vi "Legacy-monitor.vi"() -> ()   [LabVIEW 2016]
uses:
  controls/SCA states.ctl
panel:
  out "Start Sample Change":bool
  out "Rotate Wheel":bool
  out "Venting Source":bool
  out "Pumping out Source":bool
  out "insert Retract Rod":bool
  out "retract Retract Rod":bool
  out "Open Wheel GV":bool
  out "Close Wheel GV":bool
  out "insert Insert Rod":bool
  out "retract Insert Rod":bool
  out "insert Sample Rod":bool
  out "retract Sample Rod":bool
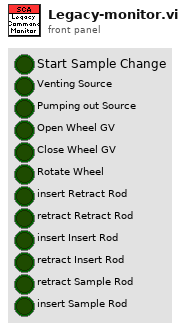
[diagram p1: front panel]
types:
  T1 = typedef "SCA states.ctl" = enum16{"initialize", "wait", "change sample start", "change sample", "check position", "rotate wheel", "sample change complete", "sample rod up", "sample rod down", "retract rod in", "retract rod out", "insert rod in", "insert rod out", "wheel GV open", "wheel GV close", "vent source", "pump source", "shutdown"}
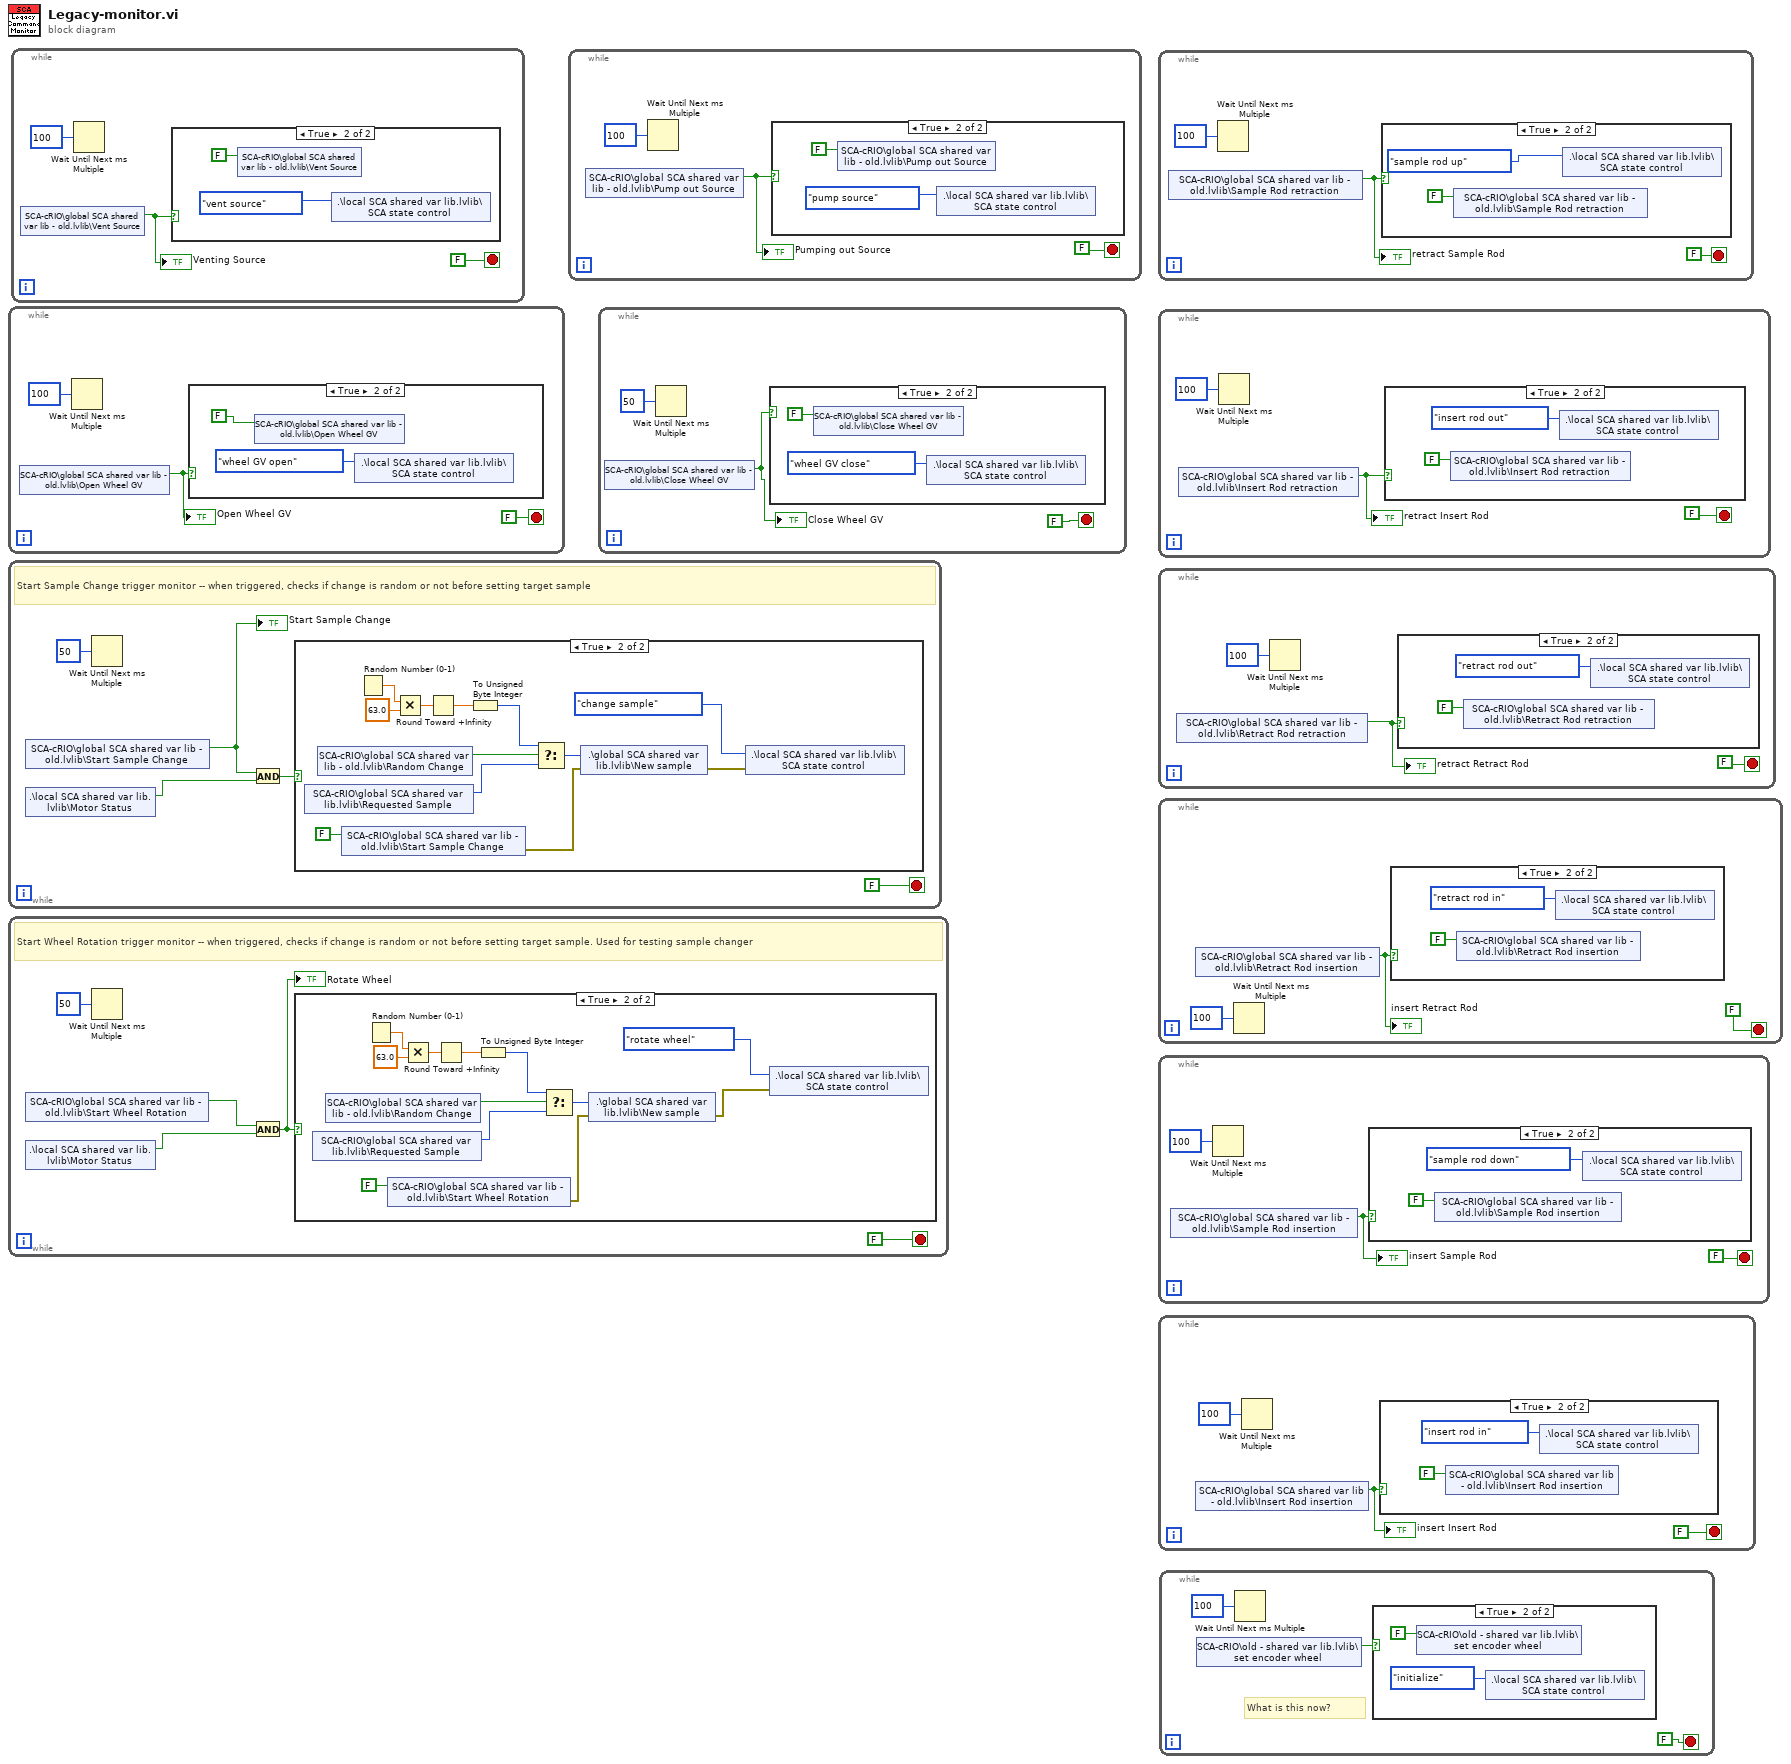
[diagram p0: block diagram]
diagram:
  n1 = while {
    stop <- FALSE stop-if-true
    n2 = shared-variable "SCA-cRIO\\global SCA shared var lib - old.lvlib\\Open Wheel GV"() -> (w2:bool)  [unwired: 1 in, 1 out]
    "Open Wheel GV" <- w2
    n3 = Wait Until Next ms Multiple(millisecond multiple=u32 100) -> ()  [unwired: 1 out]
    n4 = case shown="True" w2 {
      frame False {
      }
      frame True {
        n5 = shared-variable "SCA-cRIO\\global SCA shared var lib - old.lvlib\\Open Wheel GV"(FALSE ("rod up shared")) -> ()  [unwired: 1 in, 1 out]
        n6 = shared-variable ".\\local SCA shared var lib.lvlib\\SCA state control"(SCA_states."wheel GV open" ("SC2 state")) -> ()  [unwired: 1 in, 1 out]
      }
    }
  }
  n7 = while {
    stop <- FALSE stop-if-true
    # "Start Sample Change trigger monitor -- when triggered, checks if change is random or not before setting target sample"
    n8 = shared-variable "SCA-cRIO\\global SCA shared var lib - old.lvlib\\Start Sample Change"() -> (w8:bool)  [unwired: 1 in, 1 out]
    "Start Sample Change" <- w8
    n9 = shared-variable ".\\local SCA shared var lib.lvlib\\Motor Status"() -> (w6:bool)  [unwired: 1 in, 1 out]
    n10 = Wait Until Next ms Multiple(millisecond multiple=u32 50) -> ()  [unwired: 1 out]
    n11 = And(x=w8, y=w6) -> (x .and. y?=w7:bool)
    n12 = case shown="True" w7 {
      frame False {
      }
      frame True {
        n13 = shared-variable "SCA-cRIO\\global SCA shared var lib.lvlib\\Requested Sample"() -> (w14:u8)  [unwired: 1 in, 1 out]
        n14 = shared-variable "SCA-cRIO\\global SCA shared var lib - old.lvlib\\Random Change"() -> (w13:bool)  [unwired: 1 in, 1 out]
        n15 = shared-variable "SCA-cRIO\\global SCA shared var lib - old.lvlib\\Start Sample Change"(FALSE ("rod up shared")) -> (error out=w11:errorcluster)  [unwired: 1 in]
        n16 = Random Number (0-1)() -> (number: 0 to 1=w18:dbl)
        n17 = Multiply(x=w18, y=63.0) -> (x*y=w16:dbl)
        n18 = Round Toward +Infinity(x=w16) -> (ceil(x): smallest int >= x=w19:dbl)
        n19 = To Unsigned Byte Integer(number=w19) -> (unsigned 8bit integer=w20:u8)
        n20 = Select(t=w20, s=w13, f=w14) -> (s? t:f=w15:u8)
        n21 = shared-variable ".\\global SCA shared var lib.lvlib\\New sample"(w15, error in=w11) -> (error out=w12:errorcluster)
        n22 = shared-variable ".\\local SCA shared var lib.lvlib\\SCA state control"(SCA_states."change sample" ("SC2 state"), error in=w12) -> ()  [unwired: 1 out]
      }
    }
  }
  n23 = while {
    stop <- FALSE stop-if-true
    # "Start Wheel Rotation trigger monitor -- when triggered, checks if change is random or not before setting target sample. Used for testing sample changer"
    n24 = shared-variable "SCA-cRIO\\global SCA shared var lib - old.lvlib\\Start Wheel Rotation"() -> (w25:bool)  [unwired: 1 in, 1 out]
    n25 = shared-variable ".\\local SCA shared var lib.lvlib\\Motor Status"() -> (w24:bool)  [unwired: 1 in, 1 out]
    n26 = Wait Until Next ms Multiple(millisecond multiple=u32 50) -> ()  [unwired: 1 out]
    n27 = And(x=w25, y=w24) -> (x .and. y?=w23:bool)
    "Rotate Wheel" <- w23
    n28 = case shown="True" w23 {
      frame False {
      }
      frame True {
        n29 = shared-variable "SCA-cRIO\\global SCA shared var lib.lvlib\\Requested Sample"() -> (w31:u8)  [unwired: 1 in, 1 out]
        n30 = shared-variable "SCA-cRIO\\global SCA shared var lib - old.lvlib\\Random Change"() -> (w30:bool)  [unwired: 1 in, 1 out]
        n31 = Random Number (0-1)() -> (number: 0 to 1=w35:dbl)
        n32 = shared-variable "SCA-cRIO\\global SCA shared var lib - old.lvlib\\Start Wheel Rotation"(FALSE ("rod up shared")) -> (error out=w28:errorcluster)  [unwired: 1 in]
        n33 = Multiply(x=w35, y=63.0) -> (x*y=w33:dbl)
        n34 = Round Toward +Infinity(x=w33) -> (ceil(x): smallest int >= x=w36:dbl)
        n35 = To Unsigned Byte Integer(number=w36) -> (unsigned 8bit integer=w37:u8)
        n36 = Select(t=w37, s=w30, f=w31) -> (s? t:f=w32:u8)
        n37 = shared-variable ".\\global SCA shared var lib.lvlib\\New sample"(w32, error in=w28) -> (error out=w29:errorcluster)
        n38 = shared-variable ".\\local SCA shared var lib.lvlib\\SCA state control"(SCA_states."rotate wheel" ("SC2 state"), error in=w29) -> ()  [unwired: 1 out]
      }
    }
  }
  n39 = while {
    stop <- FALSE stop-if-true
    n40 = shared-variable "SCA-cRIO\\global SCA shared var lib - old.lvlib\\Vent Source"() -> (w41:bool)  [unwired: 1 in, 1 out]
    "Venting Source" <- w41
    n41 = Wait Until Next ms Multiple(millisecond multiple=u32 100) -> ()  [unwired: 1 out]
    n42 = case shown="True" w41 {
      frame False {
      }
      frame True {
        n43 = shared-variable "SCA-cRIO\\global SCA shared var lib - old.lvlib\\Vent Source"(FALSE ("rod up shared")) -> ()  [unwired: 1 in, 1 out]
        n44 = shared-variable ".\\local SCA shared var lib.lvlib\\SCA state control"(SCA_states."vent source" ("SCA state control")) -> ()  [unwired: 1 in, 1 out]
      }
    }
  }
  n45 = while {
    stop <- FALSE stop-if-true
    n46 = shared-variable "SCA-cRIO\\global SCA shared var lib - old.lvlib\\Pump out Source"() -> (w46:bool)  [unwired: 1 in, 1 out]
    "Pumping out Source" <- w46
    n47 = Wait Until Next ms Multiple(millisecond multiple=u32 100) -> ()  [unwired: 1 out]
    n48 = case shown="True" w46 {
      frame False {
      }
      frame True {
        n49 = shared-variable "SCA-cRIO\\global SCA shared var lib - old.lvlib\\Pump out Source"(FALSE ("rod up shared")) -> ()  [unwired: 1 in, 1 out]
        n50 = shared-variable ".\\local SCA shared var lib.lvlib\\SCA state control"(SCA_states."pump source" ("SCA state control")) -> ()  [unwired: 1 in, 1 out]
      }
    }
  }
  n51 = while {
    stop <- FALSE stop-if-true
    n52 = shared-variable "SCA-cRIO\\global SCA shared var lib - old.lvlib\\Close Wheel GV"() -> (w50:bool)  [unwired: 1 in, 1 out]
    "Close Wheel GV" <- w50
    n53 = Wait Until Next ms Multiple(millisecond multiple=u32 50) -> ()  [unwired: 1 out]
    n54 = case shown="True" w50 {
      frame False {
      }
      frame True {
        n55 = shared-variable "SCA-cRIO\\global SCA shared var lib - old.lvlib\\Close Wheel GV"(FALSE ("rod up shared")) -> ()  [unwired: 1 in, 1 out]
        n56 = shared-variable ".\\local SCA shared var lib.lvlib\\SCA state control"(SCA_states."wheel GV close" ("SC2 state")) -> ()  [unwired: 1 in, 1 out]
      }
    }
  }
  n57 = while {
    stop <- FALSE stop-if-true
    n58 = shared-variable "SCA-cRIO\\global SCA shared var lib - old.lvlib\\Sample Rod retraction"() -> (w56:bool)  [unwired: 1 in, 1 out]
    "retract Sample Rod" <- w56
    n59 = Wait Until Next ms Multiple(millisecond multiple=u32 100) -> ()  [unwired: 1 out]
    n60 = case shown="True" w56 {
      frame False {
      }
      frame True {
        n61 = shared-variable "SCA-cRIO\\global SCA shared var lib - old.lvlib\\Sample Rod retraction"(FALSE ("rod up shared")) -> ()  [unwired: 1 in, 1 out]
        n62 = shared-variable ".\\local SCA shared var lib.lvlib\\SCA state control"(SCA_states."sample rod up" ("SCA state control")) -> ()  [unwired: 1 in, 1 out]
      }
    }
  }
  n63 = while {
    stop <- FALSE stop-if-true
    n64 = shared-variable "SCA-cRIO\\global SCA shared var lib - old.lvlib\\Insert Rod retraction"() -> (w61:bool)  [unwired: 1 in, 1 out]
    "retract Insert Rod" <- w61
    n65 = Wait Until Next ms Multiple(millisecond multiple=u32 100) -> ()  [unwired: 1 out]
    n66 = case shown="True" w61 {
      frame False {
      }
      frame True {
        n67 = shared-variable "SCA-cRIO\\global SCA shared var lib - old.lvlib\\Insert Rod retraction"(FALSE ("rod up shared")) -> ()  [unwired: 1 in, 1 out]
        n68 = shared-variable ".\\local SCA shared var lib.lvlib\\SCA state control"(SCA_states."insert rod out" ("SC2 state")) -> ()  [unwired: 1 in, 1 out]
      }
    }
  }
  n69 = while {
    stop <- FALSE stop-if-true
    n70 = shared-variable "SCA-cRIO\\global SCA shared var lib - old.lvlib\\Retract Rod retraction"() -> (w66:bool)  [unwired: 1 in, 1 out]
    "retract Retract Rod" <- w66
    n71 = Wait Until Next ms Multiple(millisecond multiple=u32 100) -> ()  [unwired: 1 out]
    n72 = case shown="True" w66 {
      frame False {
      }
      frame True {
        n73 = shared-variable "SCA-cRIO\\global SCA shared var lib - old.lvlib\\Retract Rod retraction"(FALSE ("rod up shared")) -> ()  [unwired: 1 in, 1 out]
        n74 = shared-variable ".\\local SCA shared var lib.lvlib\\SCA state control"(SCA_states."retract rod out" ("SC2 state")) -> ()  [unwired: 1 in, 1 out]
      }
    }
  }
  n75 = while {
    stop <- FALSE stop-if-true
    n76 = shared-variable "SCA-cRIO\\global SCA shared var lib - old.lvlib\\Retract Rod insertion"() -> (w71:bool)  [unwired: 1 in, 1 out]
    "insert Retract Rod" <- w71
    n77 = Wait Until Next ms Multiple(millisecond multiple=u32 100) -> ()  [unwired: 1 out]
    n78 = case shown="True" w71 {
      frame False {
      }
      frame True {
        n79 = shared-variable "SCA-cRIO\\global SCA shared var lib - old.lvlib\\Retract Rod insertion"(FALSE ("rod up shared")) -> ()  [unwired: 1 in, 1 out]
        n80 = shared-variable ".\\local SCA shared var lib.lvlib\\SCA state control"(SCA_states."retract rod in" ("SC2 state")) -> ()  [unwired: 1 in, 1 out]
      }
    }
  }
  n81 = while {
    stop <- FALSE stop-if-true
    n82 = shared-variable "SCA-cRIO\\global SCA shared var lib - old.lvlib\\Sample Rod insertion"() -> (w76:bool)  [unwired: 1 in, 1 out]
    "insert Sample Rod" <- w76
    n83 = Wait Until Next ms Multiple(millisecond multiple=u32 100) -> ()  [unwired: 1 out]
    n84 = case shown="True" w76 {
      frame False {
      }
      frame True {
        n85 = shared-variable "SCA-cRIO\\global SCA shared var lib - old.lvlib\\Sample Rod insertion"(FALSE ("rod up shared")) -> ()  [unwired: 1 in, 1 out]
        n86 = shared-variable ".\\local SCA shared var lib.lvlib\\SCA state control"(SCA_states."sample rod down" ("SC2 state")) -> ()  [unwired: 1 in, 1 out]
      }
    }
  }
  n87 = while {
    stop <- FALSE stop-if-true
    n88 = shared-variable "SCA-cRIO\\global SCA shared var lib - old.lvlib\\Insert Rod insertion"() -> (w81:bool)  [unwired: 1 in, 1 out]
    "insert Insert Rod" <- w81
    n89 = Wait Until Next ms Multiple(millisecond multiple=u32 100) -> ()  [unwired: 1 out]
    n90 = case shown="True" w81 {
      frame False {
      }
      frame True {
        n91 = shared-variable "SCA-cRIO\\global SCA shared var lib - old.lvlib\\Insert Rod insertion"(FALSE ("rod up shared")) -> ()  [unwired: 1 in, 1 out]
        n92 = shared-variable ".\\local SCA shared var lib.lvlib\\SCA state control"(SCA_states."insert rod in" ("SC2 state")) -> ()  [unwired: 1 in, 1 out]
      }
    }
  }
  n93 = while {
    stop <- FALSE stop-if-true
    # "What is this now?"
    n94 = shared-variable "SCA-cRIO\\old - shared var lib.lvlib\\set encoder wheel"() -> (w85:bool)  [unwired: 1 in, 1 out]
    n95 = Wait Until Next ms Multiple(millisecond multiple=u32 100) -> ()  [unwired: 1 out]
    n96 = case shown="True" w85 {
      frame False {
      }
      frame True {
        n97 = shared-variable "SCA-cRIO\\old - shared var lib.lvlib\\set encoder wheel"(FALSE ("rod up shared")) -> ()  [unwired: 1 in, 1 out]
        n98 = shared-variable ".\\local SCA shared var lib.lvlib\\SCA state control"(SCA_states."initialize" ("SC2 state")) -> ()  [unwired: 1 in, 1 out]
      }
    }
  }
